vi "Shooter Simulator Get Bottom Limit Switch.vi"() -> (2 "Top Limit Switch":bool)   [LabVIEW 2015]
uses:
  Shooter Simulator Globals.vi
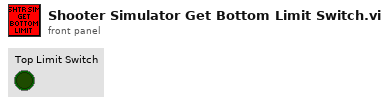
[diagram p1: front panel]
types:
  T1 = typedef "Shooter Simulator Sensor Data.ctl" = cluster{"L Enc Rate":dbl, "R Enc Rate":dbl, "Angle Encoder":dbl, "Top Limit":bool, "Bottom Limit":bool}
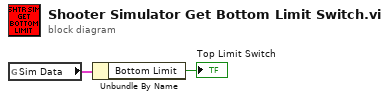
[diagram p0: block diagram]
diagram:
  n1 = global read "Shooter Simulator Globals.vi" "Sim Data"() -> (w2:T1)
  n2 = Unbundle By Name(w2) -> ("Bottom Limit"=→"Top Limit Switch":bool)
